vi "Lev-Mar Fit to encoded 2D gaussian.vi"(0 "X":dbl[](array[numeric]) format="%.2f", 1 "Standard Deviation":dbl[](array[numeric]) format="%.2f", 2 "fit type":u16, 5 "Y":dbl[](array[numeric]) format="%.2f", 7 "code":dbl format="%.3f", 9 "Initial Guess Coefficients":dbl[](array[numeric]) format="%.2f", 11 "max iteration":i32=200, 12 "derivative":T1(ring), 13 "Fit this coeff?":bool[](array[boolean])) -> (4 "Best Fit Coefficients":dbl[](array[numeric]) format="%.2f", 6 "Best Fit":dbl[](array[numeric]) format="%.2f", 8 "Covariance":dbl[][](array[numeric]) format="%.2f", 10 "mse":dbl format="%.4e", 15 "error":i32)   [LabVIEW 2016]
doc: "Uses the Levenberg-Marquardt algorithm to determine the least squares set of coefficients that best fit the set of input data points (X,Y) as expressed by a nonlinear function y=f(x,a), where a is the set of coefficients.\n\nThis subprogram is derived from a subprogram contained in the National Instruments LabView advanced analysis library. The original subprogram is copyright National Instruments."
uses:
  <vilib>/Analysis/baseanly.llb/Real Inverse Matrix.vi
  <vilib>/Analysis/NI_AALBase.lvlib
panel:
  # "Nonlinear  Lev-Mar  Fit"
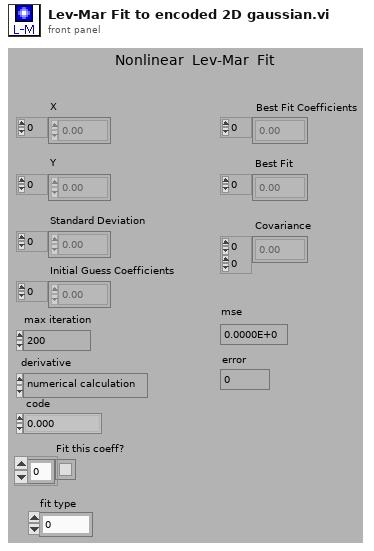
[diagram p1: front panel]
types:
  T1 = enum32{"numerical calculation", "formula calculation"}
  T2 = typedef "NI_Matrix.lvlib/RealMatrix.ctl" = dbl[][]
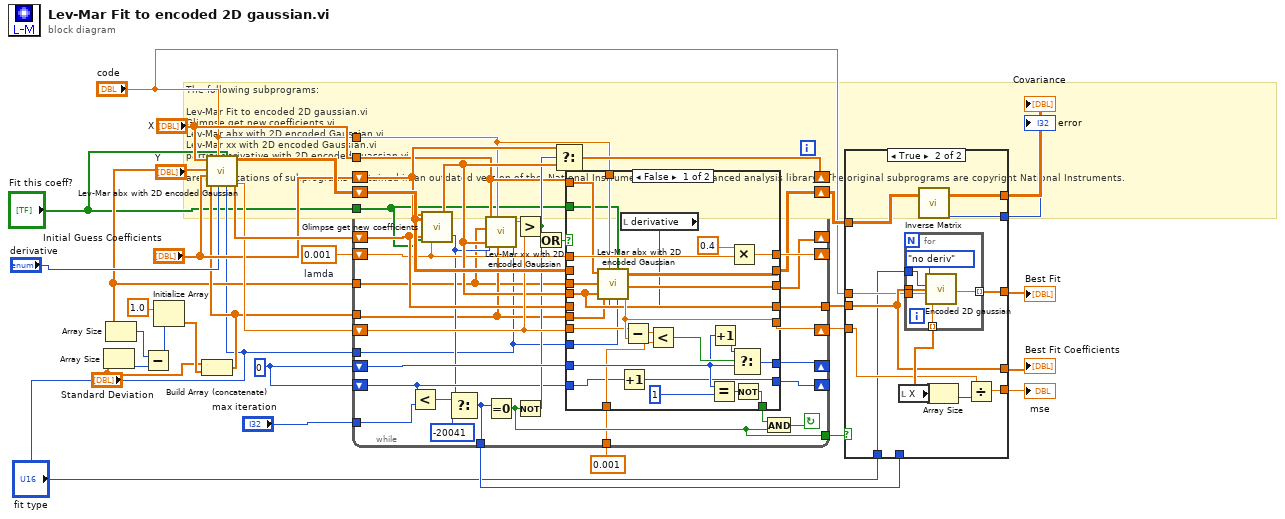
[diagram p0: block diagram]
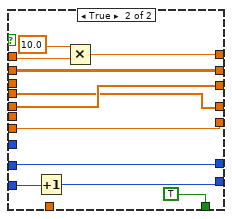
[diagram p2: hidden frame]
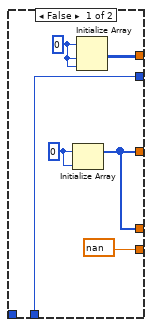
[diagram p3: hidden frame]
diagram:
  w20 = 0
  w29 = 0.001  # lamda
  # "The following subprograms:\n\nLev-Mar Fit to encoded 2D gaussian.vi\nGlimpse get new coefficients.vi\nLev-Mar abx with 2D encoded Gaussian.vi\nLev-Mar xx with 2D encoded Gaussian.vi\npartial derivative with 2D encoded guassian.vi\n\nare modifications of subprograms contained in an outdated version of the  National Instruments LabView advanced analysis library.  The original subprograms are copyright National Instruments."
  n1 = Array Size(array="Standard Deviation") -> (size(s)=w9:i32)
  n2 = Array Size(array="Y") -> (size(s)=w10:i32)
  n3 = Subtract(x=w10, y=w9) -> (x-y=w8:i32)
  n4 = Initialize Array(1.0, w8) -> (w7:dbl[])
  n5 = Build Array (concatenate)("Standard Deviation", w7) -> (w5:dbl[])
  n6 = call "Lev-Mar abx with 2D encoded Gaussian.vi"("fit type"="fit type", "Fit this coeff?"="Fit this coeff?", "derivative"="derivative", "code"="code", "Standard Deviation"=w5, "Coefficients"="Initial Guess Coefficients", "Y"="Y", "X"="X") -> ("chiSqr"=w27:dbl, "Beta"=w28:dbl[], "Alpha"=w30:dbl[][])  [unwired: 1 out]
  n7 = while {
    tunnel: "X" -> [w35]
    tunnel: "Y" -> [w37]
    tunnel: [w38] -> w12
    tunnel: "max iteration" -> [w40]
    tunnel: w5 -> [w39]
    shift-left: w20 -> [w44]
    shift-right: [w45] -> _
    tunnel: 0.001 -> [w49]
    tunnel: [w50] -> w22
    tunnel: [w53] -> w25
    shift-left: w20 -> [w58]
    shift-right: [w57] -> _
    shift-left: w27 -> [w59]
    shift-right: [w60] -> w26
    shift-left: w28 -> [w56]
    shift-right: [w61] -> _
    shift-left: w30 -> [w62]
    shift-right: [w63] -> w11
    shift-left: "Initial Guess Coefficients" -> [w36]
    shift-right: [w64] -> _
    shift-left: w29 -> [w54]
    shift-right: [w65] -> _
    tunnel: "code" -> [w34]
    tunnel: "Fit this coeff?" -> [w32]
    tunnel: "fit type" -> [w33]
    stop <- w52 continue-if-true
    n8 = Less?(x=w44, y=w40) -> (x < y?=w43:bool)
    n9 = call "Glimpse get new coefficients.vi"("Coefficients"=w36, "Alpha"=w62, "Beta"=w56, "Fit this coeff?"=w32, "lamda"=w54) -> ("New Coefficients"=w55:dbl[], "error"=w41:i32)  [unwired: 9 out]
    n10 = Select(t=w41, s=w43, f=-20041) -> (s? t:f=w38:i32)
    n11 = call "Lev-Mar xx with 2D encoded Gaussian.vi"("fit type"=w33, "Standard Deviation"=w39, "code"=w34, "error"=w41, "Coefficients"=w55, "Y"=w37, "X"=w35) -> ("chiSqr"=w66:dbl)  [unwired: 3 out]
    n12 = Equal To 0?(x=w38) -> (x = 0?=w50:bool)
    n13 = Greater?(x=w66, y=w59) -> (0:w47:bool)
    n14 = Not(x=w50) -> (.not. x?=w46:bool)
    n15 = Or(x=w47, y=w46) -> (x .or. y?=w48:bool)
    n16 = Select(t=w36, s=w47, f=w55) -> (s? t:f=w64:dbl[])
    n17 = case shown="False" w48 {
      tunnel: w54 -> [w91 w102]
      tunnel: [w90 w101] -> w65
      tunnel: [w89 w100] -> w63
      tunnel: w62 -> [_ w100]
      tunnel: [w88 w96] -> w61
      tunnel: [w87 w99] -> w60
      tunnel: w59 -> [w86 w99]
      tunnel: w58 -> [w81 w98]
      tunnel: [w82 w98] -> w57
      tunnel: [w78 TRUE] -> w51
      tunnel: w55 -> [w75 w95]
      tunnel: w56 -> [_ w96]
      tunnel: [w75 w95] -> w53
      tunnel: w49 -> [w77 _]
      tunnel: [w72 w94] -> w45
      tunnel: w44 -> [w76 w93]
      tunnel: w39 -> [w74 _]
      tunnel: w35 -> [w71 _]
      tunnel: w37 -> [w70 _]
      tunnel: w34 -> [w69 _]
      tunnel: w33 -> [w68 _]
      tunnel: w32 -> [w67 _]
      frame False {
        n18 = Increment(x=w76) -> (x+1=w72:i32)
        n19 = local read "derivative"() -> (w73:T1)
        n20 = call "Lev-Mar abx with 2D encoded Gaussian.vi"("fit type"=w68, "Fit this coeff?"=w67, "derivative"=w73, "code"=w69, "Standard Deviation"=w74, "Coefficients"=w75, "Y"=w70, "X"=w71) -> ("chiSqr"=w87:dbl, "Beta"=w88:dbl[], "Alpha"=w89:dbl[][])  [unwired: 1 out]
        n21 = Subtract(x=w86, y=w87) -> (x-y=w85:dbl)
        n22 = Less?(x=w85, y=w77) -> (x < y?=w84:bool)
        n23 = Equal?(x=w81, y=1) -> (x = y?=w79:bool)
        n24 = Increment(x=w81) -> (x+1=w83:i32)
        n25 = Multiply(x=0.4, y=w91) -> (x*y=w90:dbl)
        n26 = Select(t=w83, s=w84, f=w81) -> (s? t:f=w82:i32)
        n27 = Not(x=w79) -> (.not. x?=w78:bool)
      }
      frame True {
        n28 = Increment(x=w93) -> (x+1=w94:i32)
        n29 = Multiply(x=10.0, y=w102) -> (x*y=w101:dbl)
      }
    }
    n30 = And(x=w51, y=w50) -> (x .and. y?=w52:bool)
  }
  n31 = case shown="True" w22 {
    tunnel: w25 -> [_ w116]
    tunnel: [w107 w116] -> w24
    tunnel: [nan w120] -> w23
    tunnel: [w107 w117] -> w15
    tunnel: w26 -> [_ w115]
    tunnel: [w105 w114] -> w14
    tunnel: [w104 w113] -> w13
    tunnel: w12 -> [w104 _]
    tunnel: w11 -> [_ w112]
    tunnel: "code" -> [_ w111]
    tunnel: "fit type" -> [_ w110]
    frame False {
      w106 = 0
      w109 = 0
      n32 = Initialize Array(w109, w109) -> (w107:i32[])
      n33 = Initialize Array(w106, w106, w106) -> (w105:i32[][])
    }
    frame True {
      n34 = local read "X"() -> (w119:dbl[])
      n35 = for {
        tunnel: w116 -> [w125]
        tunnel: [w124] -> w117 mode=indexing
        tunnel: w119 -> [w126] mode=indexing
        tunnel: w111 -> [w122]
        tunnel: w110 -> [w121]
        n36 = call "Encoded 2D gaussian.vi"("Coefficients"=w125, "X"=w126, "code"=w122, "fit type"=w121, "Flag"=enum16{"no deriv", "deriv"}."no deriv") -> ("Y"=w124:dbl)  [unwired: 4 out]
      }
      n37 = call-poly <vilib>:"Inverse Matrix.vi"("Input Matrix"=w112) -> ("error"=w113:i32, "Inverse Matrix"=w114:T2)  [unwired: 1 in]
      n38 = Array Size(array=w119) -> (size(s)=w118:i32)
      n39 = Divide(x=w115, y=w118) -> (x/y=w120:dbl)
    }
  }
  "mse" <- w23
  "Best Fit Coefficients" <- w24
  "Best Fit" <- w15
  "error" <- w13
  "Covariance" <- w14
